vi "PID Control.vi"(8 "error in (no error)":errorcluster, 11 "Data":T1) -> ()   [LabVIEW 2020]
uses:
  <vilib>/numeric/Random Number (Range) DBL.vi
  <vilib>/addons/control/pid/pid.llb/PID (DBL).vi
  <vilib>/addons/control/pid/NI_PID_pid.lvlib
  <userlib>/_OpenG.lib/time/time.llb/openg_time.lvlib
panel:
  out "PID Controller":T2(graph)
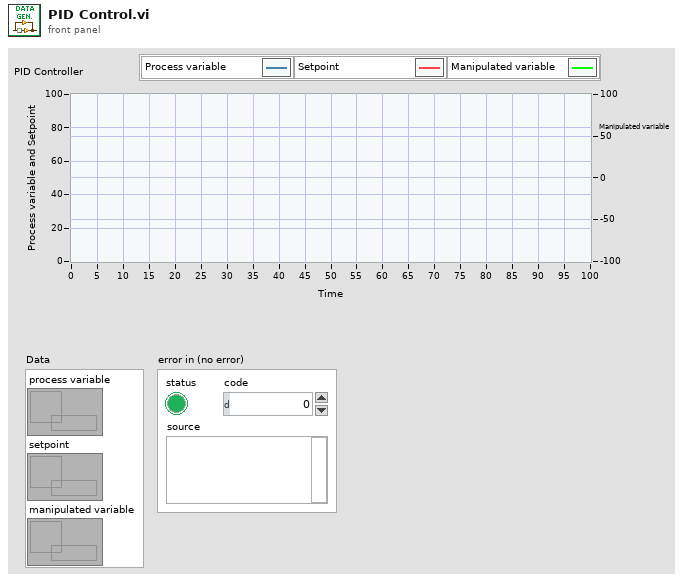
[diagram p1: front panel]
types:
  T1 = cluster{"process variable":refnum<queue>, "setpoint":refnum<queue>, "manipulated variable":refnum<queue>}
  T2 = cluster{"Plant Output":dbl, "number":dbl, "output":dbl}
  T3 = cluster{"proportional gain (Kc)":dbl, "integral time (Ti, min)":dbl, "derivative time (Td, min)":dbl}
  T4 = cluster{"channel":string, "current time":timestamp, "data":dbl}
  T5 = cluster{"static gain":dbl, "lag (min)":dbl, "dead cycles":dbl, "load %":dbl, "deadband":dbl, "noise level %":dbl, "initial PV":dbl, "initial PV 2":dbl}
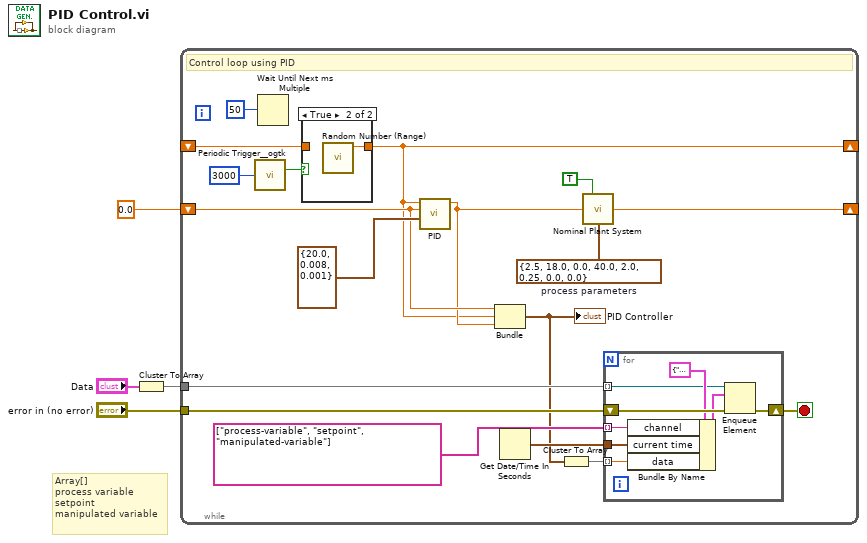
[diagram p0: block diagram]
diagram:
  # "Array[]\nprocess variable\nsetpoint\nmanipulated variable"
  n1 = Cluster To Array(cluster="Data") -> (array=w1:refnum<queue>[])
  n2 = while {
    shift-left: 0.0 ("Plant Output") -> [w14]
    shift-right: [w22] -> _
    shift-right: [w8] -> _
    shift-left: _ -> [w16]
    tunnel: w1 -> [w6]
    tunnel: "error in (no error)" -> [w10]
    stop <- w7 stop-if-true
    w20 = T5 {"static gain"=2.5, "lag (min)"=18.0, "dead cycles"=0.0, "load %"=40.0, "deadband"=2.0, "noise level %"=0.25, "initial PV"=0.0, "initial PV 2"=0.0}  # process parameters
    # "Control loop using PID"
    n3 = call <userlib>:"Periodic Trigger__ogtk.vi"("time (ms)"=u32 3000) -> ("Triggered"=w17:bool)  [unwired: 12 in, 2 out]
    n4 = Wait Until Next ms Multiple(millisecond multiple=u32 50 ("unsigned 32bit integer")) -> ()  [unwired: 1 out]
    n5 = case shown="True" w17 {
      tunnel: [w31 w32] -> w8
      tunnel: w16 -> [w31 _]
      frame False {
      }
      frame True {
        n6 = call-poly <vilib>:"Random Number (Range).vi"() -> ("number"=w32:dbl)  [unwired: 11 in]
      }
    }
    n7 = call-poly <vilib>:"PID.vi"("PID gains"=T3 {"proportional gain (Kc)"=20.0, "integral time (Ti, min)"=0.008, "derivative time (Td, min)"=0.001}, "process variable"=w14, "setpoint"=w8) -> ("output"=w13:dbl)  [unwired: 7 in, 1 out]
    n8 = Bundle("Plant Output"=w14, "number"=w8, "output"=w13) -> (w5:T2)  [unwired: 1 in]
    "PID Controller" <- w5
    n9 = Get Date/Time In Seconds() -> (seconds since 1Jan1904=w9:timestamp)
    n10 = Cluster To Array(cluster=w5) -> (array=w11:dbl[])
    n11 = call "Nominal Plant System.vi"("Integrator ?"=TRUE, "Plant Input"=w13, "process parameters"=w20) -> ("Plant Output"=w22:dbl)  [unwired: 12 in]
    n12 = for {
      tunnel: string[] ["process-variable", "setpoint", "manipulated-variable"] -> [w30] mode=indexing
      tunnel: w9 -> [w29]
      tunnel: w11 -> [w28] mode=indexing
      shift-right: [w27] -> w7
      shift-left: w10 -> [w26]
      tunnel: w6 -> [w23] mode=indexing
      n13 = Bundle By Name(cluster=T4 {"channel"="", "current time"=timestamp(0 s since 1904-01-01), "data"=0.0} ("element"), "channel"=w30, "current time"=w29, "data"=w28) -> (w24:T4)
      n14 = Enqueue Element(queue=w23, element=w24, error in (no error)=w26) -> (error out=w27:errorcluster)  [unwired: 1 in, 2 out]
    }
  }
